vi "Apply Configuration Maxima and Minima to Facade Controls.vi"(10 "references":T1, 11 "Display State In":T2) -> (3 "Display State Out":T2)   [LabVIEW 2017, in "Test Signal Configuration.xctl"]
uses:
  <vilib>/addons/_XControls/Function Generator Configuration/Test Signal Configuration.xctl
  <vilib>/addons/_XControls/Function Generator Configuration/Controls/State.ctl
  <vilib>/addons/_XControls/Function Generator Configuration/Controls/references.ctl
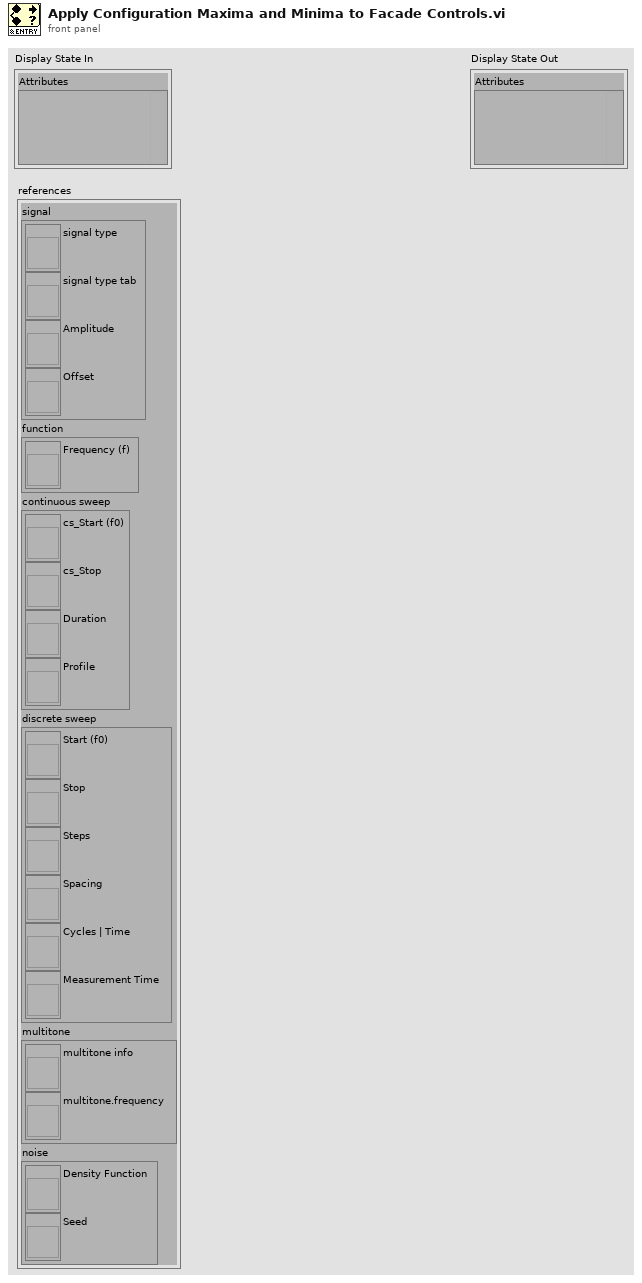
[diagram p1: front panel]
types:
  T1 = typedef "Test Signal Configuration.xctl/references.ctl" = cluster{"signal":cluster{"signal type":refnum<vi>, "signal type tab":refnum<vi>, "Amplitude":refnum<vi>, "Offset":refnum<vi>}, "function":cluster{"Frequency (f)":refnum<vi>}, "continuous sweep":cluster{"cs_Start (f0)":refnum<vi>, "cs_Stop":refnum<vi>, "Duration":refnum<vi>, "Profile":refnum<vi>}, "discrete sweep":cluster{"Start (f0)":refnum<vi>, "Stop":refnum<vi>, "Steps":refnum<vi>, "Spacing":refnum<vi>, "Cycles | Time":refnum<vi>, "Measurement Time":refnum<vi>}, "multitone":cluster{"multitone info":refnum<vi>, "multitone.frequency":refnum<vi>}, "noise":cluster{"Density Function":refnum<vi>, "Seed":refnum<vi>}}
  T2 = typedef "Test Signal Configuration.xctl/State.ctl" = cluster{"Attributes":variant}
  T3 = cluster{"frequency":dbl, "amplitude":dbl, "phase":dbl}[]
  T4 = cluster{"frequency":dbl, "amplitude":dbl, "phase":dbl}
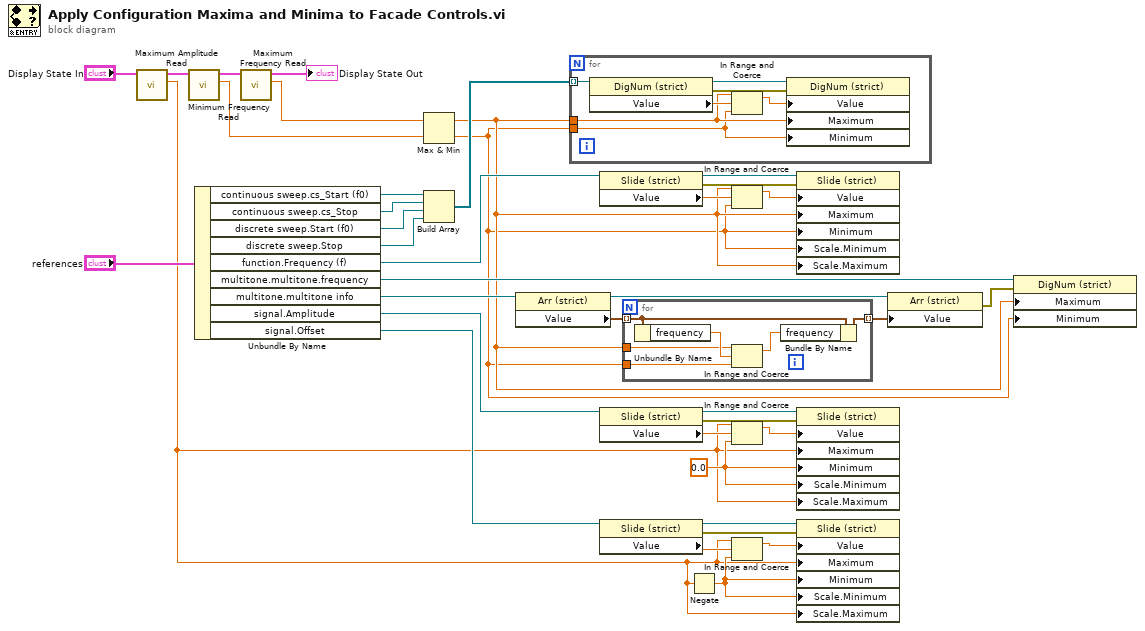
[diagram p0: block diagram]
diagram:
  w10 = 0.0 ("lower limit")
  n1 = call <vilib>:"Maximum Amplitude Read.vi"("Display State In"="Display State In") -> ("Value"=w1:dbl, "Display State Out"=w6:T2)  [unwired: 4 in, 1 out]
  n2 = call <vilib>:"Minimum Frequency Read.vi"("Display State In"=w6) -> ("Value"=w2:dbl, "Display State Out"=w5:T2)  [unwired: 4 in, 1 out]
  n3 = Unbundle By Name("references") -> ("continuous sweep.cs_Start (f0)"=w37:refnum<vi>, "continuous sweep.cs_Stop"=w36:refnum<vi>, "discrete sweep.Start (f0)"=w35:refnum<vi>, "discrete sweep.Stop"=w34:refnum<vi>, "function.Frequency (f)"=w23:refnum<vi>, "multitone.multitone.frequency"=w25:refnum<vi>, "multitone.multitone info"=w24:refnum<vi>, "signal.Amplitude"=w19:refnum<vi>, "signal.Offset"=w12:refnum<vi>)
  n4 = call <vilib>:"Maximum Frequency Read.vi"("Display State In"=w5) -> ("Value"=w3:dbl, "Display State Out"=→"Display State Out":T2)  [unwired: 4 in, 1 out]
  n5 = Max & Min(x=w3, y=w2) -> (max(x,y)=w9:dbl, min(x,y)=w8:dbl)
  n6 = Build Array(w37, w36, w35, w34) -> (w33:refnum<vi>[])
  n7 = property class="Arr (strict)"(reference=w24) -> (reference out=w29:refnum<vi>, "Value"=w28:T3)  [unwired: 1 in, 1 out]
  n8 = for {
    tunnel: w33 -> [w45] mode=indexing
    tunnel: w9 -> [w42]
    tunnel: w8 -> [w41]
    n9 = property class="DigNum (strict)"(reference=w45) -> (reference out=w40:refnum<vi>, error out=w39:errorcluster, "Value"=w44:dbl)  [unwired: 1 in]
    n10 = In Range and Coerce(upper limit=w42, x=w44, lower limit=w41) -> (coerced(x)=w43:dbl)  [unwired: 1 out]
    n11 = property class="DigNum (strict)"(reference=w40, error in=w39, "Value"=w43, "Maximum"=w42, "Minimum"=w41) -> ()  [unwired: 2 out]
  }
  n12 = property class="Slide (strict)"(reference=w23) -> (reference out=w30:refnum<vi>, error out=w17:errorcluster, "Value"=w31:dbl)  [unwired: 1 in]
  n13 = property class="Slide (strict)"(reference=w19) -> (reference out=w22:refnum<vi>, error out=w18:errorcluster, "Value"=w21:dbl)  [unwired: 1 in]
  n14 = property class="Slide (strict)"(reference=w12) -> (reference out=w13:refnum<vi>, error out=w16:errorcluster, "Value"=w14:dbl)  [unwired: 1 in]
  n15 = for {
    tunnel: w28 -> [w46] mode=indexing
    tunnel: w9 -> [w50]
    tunnel: w8 -> [w49]
    tunnel: [w47] -> w26 mode=indexing
    n16 = Unbundle By Name(w46) -> ("frequency"=w51:dbl)
    n17 = In Range and Coerce(upper limit=w50, x=w51, lower limit=w49) -> (coerced(x)=w48:dbl)  [unwired: 1 out]
    n18 = Bundle By Name(cluster=w46, "frequency"=w48) -> (w47:T4)
  }
  n19 = Negate(x=w1) -> (-x=w11:dbl)
  n20 = In Range and Coerce(upper limit=w9, x=w31, lower limit=w8) -> (coerced(x)=w32:dbl)  [unwired: 1 out]
  n21 = In Range and Coerce(upper limit=w1, x=w21, lower limit=w10) -> (coerced(x)=w20:dbl)  [unwired: 1 out]
  n22 = In Range and Coerce(upper limit=w1, x=w14, lower limit=w11) -> (coerced(x)=w15:dbl)  [unwired: 1 out]
  n23 = property class="Slide (strict)"(reference=w30, error in=w17, "Value"=w32, "Maximum"=w9, "Minimum"=w8, "Scale.Minimum"=w8, "Scale.Maximum"=w9) -> ()  [unwired: 2 out]
  n24 = property class="Slide (strict)"(reference=w22, error in=w18, "Value"=w20, "Maximum"=w1, "Minimum"=w10, "Scale.Minimum"=w10, "Scale.Maximum"=w1) -> ()  [unwired: 2 out]
  n25 = property class="Slide (strict)"(reference=w13, error in=w16, "Value"=w15, "Maximum"=w1, "Minimum"=w11, "Scale.Minimum"=w11, "Scale.Maximum"=w1) -> ()  [unwired: 2 out]
  n26 = property class="Arr (strict)"(reference=w29, "Value"=w26) -> (error out=w27:errorcluster)  [unwired: 1 in, 1 out]
  n27 = property class="DigNum (strict)"(reference=w25, error in=w27, "Maximum"=w9, "Minimum"=w8) -> ()  [unwired: 2 out]
